vi "Create Tool String.vi"(11 "Tool":T1) -> (3 "String":string)   [LabVIEW 2025, in "Tools.lvlib" / "PyServer.lvclass"]
uses:
  PyServer.lvclass
  Toolset.ctl
  Datatypes.ctl
  PyServer.lvclass/PyServer.ctl
  Tools.lvlib
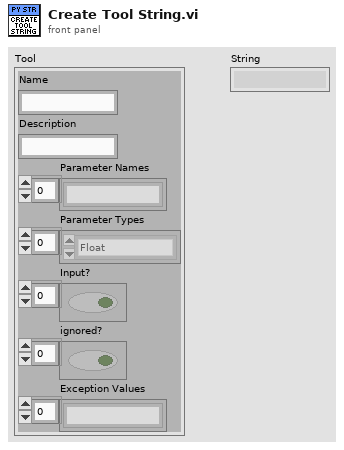
[diagram p1: front panel]
types:
  T1 = typedef "Tools.lvlib/PyServer.lvclass/Toolset.ctl" = cluster{"Name":string, "Description":string, "Parameter Names":string[], "Parameter Types":T2[], "Input?":bool[], "ignored?":bool[], "Exception Values":string[]}
  T2 = typedef "Tools.lvlib/Datatypes.ctl" = enum16{"Float", "Int", "String", "String Array", "Int Array", "Float Array", "Bool Array", "Bool", "Invalid"}
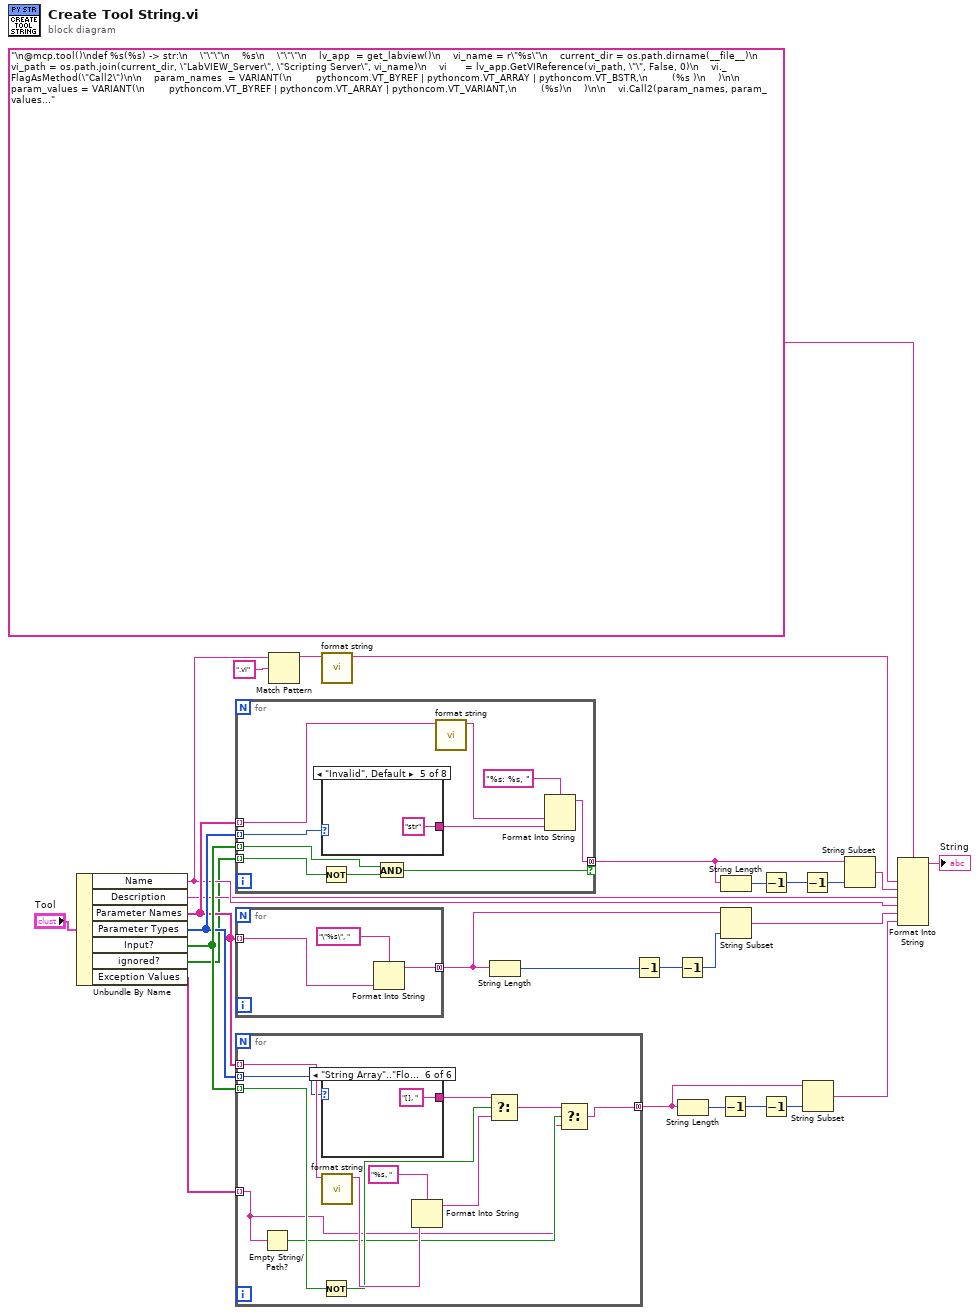
[diagram p0: block diagram]
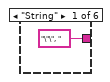
[diagram p2: hidden frame]
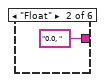
[diagram p3: hidden frame]
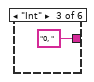
[diagram p4: hidden frame]
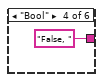
[diagram p5: hidden frame]
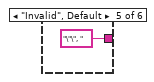
[diagram p6: hidden frame]
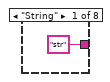
[diagram p7: hidden frame]
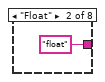
[diagram p8: hidden frame]
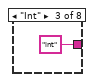
[diagram p9: hidden frame]
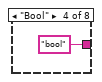
[diagram p10: hidden frame]
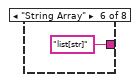
[diagram p11: hidden frame]
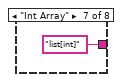
[diagram p12: hidden frame]
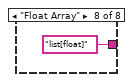
[diagram p13: hidden frame]
diagram:
  n1 = Unbundle By Name("Tool") -> ("Name"=w13:string, "Description"=w12:string, "Parameter Names"=w24:string[], "Parameter Types"=w25:T2[], "Input?"=w28:bool[], "ignored?"=w6:bool[], "Exception Values"=w1:string[])
  n2 = for {
    tunnel: w24 -> [w30] mode=indexing
    tunnel: w28 -> [w38] mode=indexing
    tunnel: [w34] -> w10 mode=concatenating if=w33
    tunnel: w25 -> [w37] mode=indexing
    tunnel: w6 -> [w32] mode=indexing
    n3 = Not(x=w32) -> (.not. x?=w31:bool)
    n4 = case shown="\"Invalid\", Default" w37 {
      tunnel: ["str" ("format string") "float" ("format string") "int" ("format string") "bool" ("format string") "str" ("format string") "list[str]" ("format string") "list[int]" ("format string") "list[float]" ("format string")] -> w35
      frame "String" {
      }
      frame "Float" {
      }
      frame "Int" {
      }
      frame "Bool" {
      }
      frame "Invalid", Default {
      }
      frame "String Array" {
      }
      frame "Int Array" {
      }
      frame "Float Array" {
      }
    }
    n5 = And(x=w38, y=w31) -> (x .and. y?=w33:bool)
    n6 = call "format string.vi"("Label.Text"=w30) -> ("String"=w29:string)  [unwired: 10 in]
    n7 = Format Into String(format string="%s: %s, ", w29, w35) -> (resulting string=w34:string)  [unwired: 2 in, 1 out]
  }
  n8 = for {
    tunnel: [w48] -> w18 mode=concatenating
    tunnel: w24 -> [w47] mode=indexing
    n9 = Format Into String(format string="\"%s\", ", w47) -> (resulting string=w48:string)  [unwired: 2 in, 1 out]
  }
  n10 = for {
    tunnel: [w52] -> w20 mode=concatenating
    tunnel: w24 -> [w60] mode=indexing
    tunnel: w25 -> [w59] mode=indexing
    tunnel: w28 -> [w54] mode=indexing
    tunnel: w1 -> [w50] mode=indexing
    n11 = Empty String/Path?(string/path=w50) -> (empty?=w51:bool)
    n12 = Not(x=w54) -> (.not. x?=w53:bool)
    n13 = case shown="\"String Array\"..\"Float Array\"" w59 {
      tunnel: ["\"\", " ("format string") "0.0, " ("format string") "0, " ("format string") "False, " ("format string") "\"\", " ("format string") "[], " ("format string")] -> w58
      frame "String" {
      }
      frame "Float" {
      }
      frame "Int" {
      }
      frame "Bool" {
      }
      frame "Invalid", Default {
      }
      frame "String Array".."Float Array" {
      }
    }
    n14 = call "format string.vi"("Label.Text"=w60) -> ("String"=w57:string)  [unwired: 10 in]
    n15 = Format Into String(format string="%s, ", w57) -> (resulting string=w55:string)  [unwired: 2 in, 1 out]
    n16 = Select(t=w58, s=w53, f=w55) -> (s? t:f=w61:string)
    n17 = Select(t=w61, s=w51, f=w50) -> (s? t:f=w52:string)
  }
  n18 = Match Pattern(string=w13, regular expression=".vi") -> (before substring=w3:string)  [unwired: 1 in, 3 out]
  n19 = call "format string.vi"("Label.Text"=w3) -> ("String"=w14:string)  [unwired: 10 in]
  n20 = String Length(string=w18) -> (length=w16:i32)
  n21 = Decrement(x=w16) -> (x-1=w17:i32)
  n22 = Decrement(x=w17) -> (x-1=w15:i32)
  n23 = String Length(string=w20) -> (length=w22:i32)
  n24 = Decrement(x=w22) -> (x-1=w21:i32)
  n25 = String Length(string=w10) -> (length=w8:i32)
  n26 = String Subset(string=w18, length (rest)=w15) -> (substring=w19:string)  [unwired: 1 in]
  n27 = Decrement(x=w8) -> (x-1=w9:i32)
  n28 = Decrement(x=w21) -> (x-1=w23:i32)
  n29 = Decrement(x=w9) -> (x-1=w7:i32)
  n30 = String Subset(string=w20, length (rest)=w23) -> (substring=w26:string)  [unwired: 1 in]
  n31 = String Subset(string=w10, length (rest)=w7) -> (substring=w11:string)  [unwired: 1 in]
  n32 = Format Into String(format string="\n@mcp.tool()\ndef %s(%s) -> str:\n    \"\"\"\n    %s\n    \"\"\"\n    lv_app  = get_labview()\n    vi_name = r\"%s\"\n    current_dir = os.path.dirname(__file__)\n    vi_path = os.path.join(current_dir, \"LabVIEW_Server\", \"Scripting Server\", vi_name)\n    vi      = lv_app.GetVIReference(vi_path, \"\", False, 0)\n    vi._FlagAsMethod(\"Call2\")\n\n    param_names  = VARIANT(\n        pythoncom.VT_BYREF | pythoncom.VT_ARRAY | pythoncom.VT_BSTR,\n        (%s )\n    )\n\n    param_values = VARIANT(\n        pythoncom.VT_BYREF | pythoncom.VT_ARRAY | pythoncom.VT_VARIANT,\n        (%s)\n    )\n\n    vi.Call2(param_names, param_values,\n            False,   # open FP?\n            False,   # close FP after call?\n            False,   # suspend on call?\n            False)   # bring LabVIEW to front?\n    \n    return param_values\n\n", w14, w11, w12, w13, w19, w26) -> (resulting string=→"String":string)  [unwired: 2 in, 1 out]
